vi "Decode_data.vi"(2 "data size":i32, 3 "Channel 1 data":u8[](array[numeric]), 4 "Channel 0 data":u8[](array[numeric])) -> (0 "Data HEX":u16[](array[numeric]), 1 "Converted data":dbl[](array[numeric]))   [LabVIEW 2010]
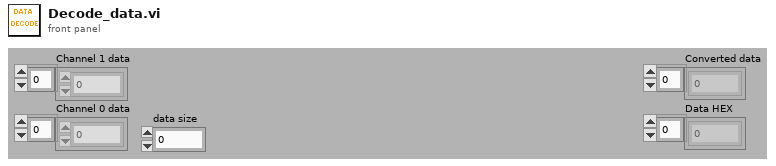
[diagram p1: front panel]
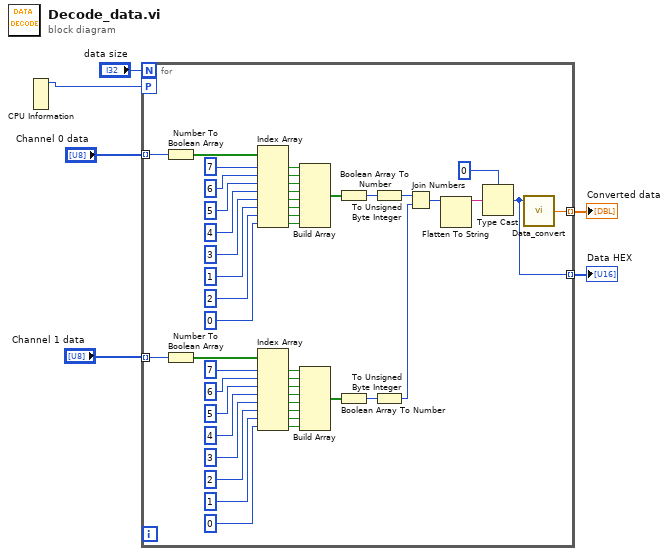
[diagram p0: block diagram]
diagram:
  n1 = CPU Information() -> (4:w5:i32)  [unwired: 3 out]
  n2 = for {
    N: "data size" -> [_]
    tunnel: "Channel 0 data" -> [w15] mode=indexing
    tunnel: "Channel 1 data" -> [w14] mode=indexing
    tunnel: [w8] -> w2 mode=indexing
    workers-P: w5 -> [_]
    tunnel: [w7] -> w1 mode=indexing
    n3 = Number To Boolean Array(number=w15) -> (Boolean array=w17:bool[])
    n4 = Number To Boolean Array(number=w14) -> (Boolean array=w16:bool[])
    n5 = Index Array(array=w17, index #1=7 ("index"), index #2=6 ("index"), index #3=5 ("index"), index #4=4 ("index"), index #5=3 ("index"), index #6=1 ("index"), index #7=2 ("index"), index #8=0 ("index")) -> (element #1=w37:bool, element #2=w36:bool, element #3=w35:bool, element #4=w34:bool, element #5=w23:bool, element #6=w22:bool, element #7=w21:bool, element #8=w20:bool)
    n6 = Index Array(array=w16, index #1=7 ("index"), index #2=6 ("index"), index #3=5 ("index"), index #4=4 ("index"), index #5=3 ("index"), index #6=2 ("index"), index #7=1 ("index"), index #8=0 ("index")) -> (element #1=w31:bool, element #2=w30:bool, element #3=w29:bool, element #4=w28:bool, element #5=w27:bool, element #6=w26:bool, element #7=w25:bool, element #8=w24:bool)
    n7 = Build Array(w37, w36, w35, w34, w23, w22, w21, w20) -> (w33:bool[])
    n8 = Build Array(w31, w30, w29, w28, w27, w26, w25, w24) -> (w32:bool[])
    n9 = Boolean Array To Number(Boolean array=w33) -> (number=w18:u32)
    n10 = Boolean Array To Number(Boolean array=w32) -> (number=w19:u32)
    n11 = To Unsigned Byte Integer(number=w18) -> (unsigned 8bit integer=w12:u8)
    n12 = To Unsigned Byte Integer(number=w19) -> (unsigned 8bit integer=w13:u8)
    n13 = Join Numbers(hi=w12, lo=w13) -> ((hi.lo)=w9:u16)
    n14 = Flatten To String(anything=w9) -> (data string=w10:string)  [unwired: 3 in, 2 out]
    n15 = Type Cast(type=u16 0, x=w10) -> (*(type *) &x=w7:u16)
    n16 = call "Data_convert.vi"("Channel data"=w7) -> ("Converted data"=w8:dbl)  [unwired: 2 in]
  }
  "Converted data" <- w2
  "Data HEX" <- w1
